vi "Configure Measurement (Spectrum Emissions Mask).vi"(0 "VISA resource name":refnum<visa-resource-name>, 5 "Measurement Type (0: Total Power Reference)":i32(ring) items=["Total Power Reference", "PSD Reference", "Spectrum Peak Reference"], 7 "Auto Power Reference (T: Enable)":bool=TRUE, 9 "Manual Reference Power (0 dBm)":dbl format="%#.6g", 11 "error in (no error)":errorcluster) -> (4 "VISA resource name out":refnum<visa-resource-name>, 15 "error out":errorcluster)   [LabVIEW 2014, in "Agilent MXA Series.lvlib"]
doc: "Sets the Spectrum Emission Mask measurement parameters."
uses:
  Agilent MXA Series.lvlib
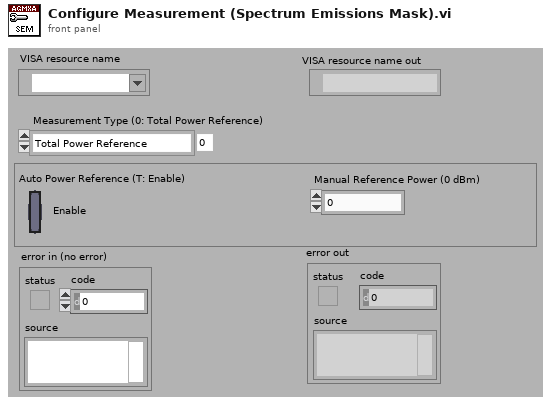
[diagram p1: front panel]
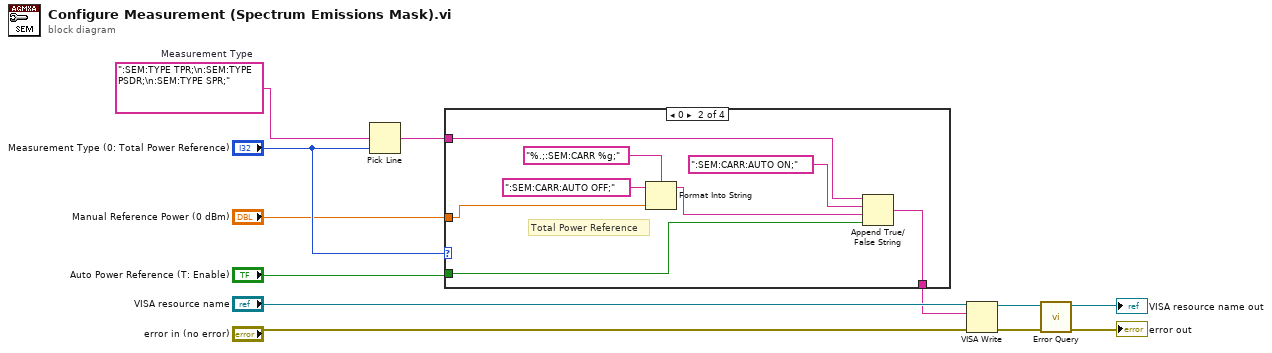
[diagram p0: block diagram]
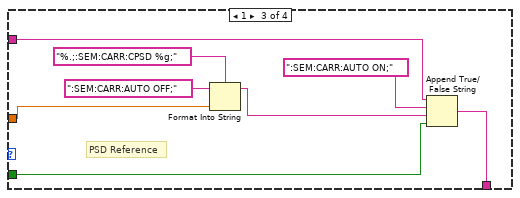
[diagram p3: hidden frame]
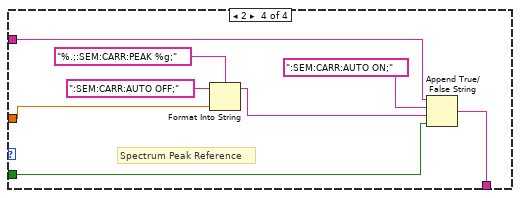
[diagram p4: hidden frame]
diagram:
  w12 = ":SEM:TYPE TPR;\n:SEM:TYPE PSDR;\n:SEM:TYPE SPR;"  # Measurement Type
  n1 = Pick Line(multi-line string=w12, line index="Measurement Type (0: Total Power Reference)") -> (output string=w1:string)  [unwired: 1 in]
  n2 = case shown="0" "Measurement Type (0: Total Power Reference)" {
    tunnel: "Auto Power Reference (T: Enable)" -> [_ w18 w26 w34]
    tunnel: "Manual Reference Power (0 dBm)" -> [_ w21 w29 w37]
    tunnel: w1 -> [w13 w16 w24 w32]
    tunnel: [w13 w14 w22 w30] -> w6
    frame Default {
    }
    frame 0 {
      # "Total Power Reference"
      n3 = Format Into String(format string="%.;:SEM:CARR %g;", initial string=":SEM:CARR:AUTO OFF;", w21) -> (resulting string=w15:string)  [unwired: 1 in, 1 out]
      n4 = Append True/False String(1:w18, 2:w15, 3:":SEM:CARR:AUTO ON;" ("true string"), 4:w16) -> (0:w14:string)
    }
    frame 1 {
      # "PSD Reference"
      n5 = Format Into String(format string="%.;:SEM:CARR:CPSD %g;", initial string=":SEM:CARR:AUTO OFF;", w29) -> (resulting string=w23:string)  [unwired: 1 in, 1 out]
      n6 = Append True/False String(1:w26, 2:w23, 3:":SEM:CARR:AUTO ON;" ("true string"), 4:w24) -> (0:w22:string)
    }
    frame 2 {
      # "Spectrum Peak Reference"
      n7 = Format Into String(format string="%.;:SEM:CARR:PEAK %g;", initial string=":SEM:CARR:AUTO OFF;", w37) -> (resulting string=w31:string)  [unwired: 1 in, 1 out]
      n8 = Append True/False String(1:w34, 2:w31, 3:":SEM:CARR:AUTO ON;" ("true string"), 4:w32) -> (0:w30:string)
    }
  }
  n9 = VISA Write(VISA resource name="VISA resource name", write buffer=w6, error in (no error)="error in (no error)") -> (VISA resource name out=w4:refnum<visa-resource-name>, error out=w5:errorcluster)  [unwired: 1 out]
  n10 = call "Error Query.vi"("error in (no error)"=w5, "VISA resource name"=w4) -> ("error out"=→"error out":errorcluster, "VISA resource name out"=→"VISA resource name out":refnum<visa-resource-name>)  [unwired: 6 in, 2 out]
